vi "VSM9T_Queue_Commands.vi"(1 "VSM-9T-Control-Cluster":T1 {"Rate (T/min)" format="%6_5f"}, 3 "15T Queue":refnum<queue>) -> (0 "VSM-9T-Control-Cluster new Status":T1 {"Rate (T/min)" format="%6_5f"})   [LabVIEW 2019]
uses:
  VSM/VSM9T-Control-Cluster.ctl
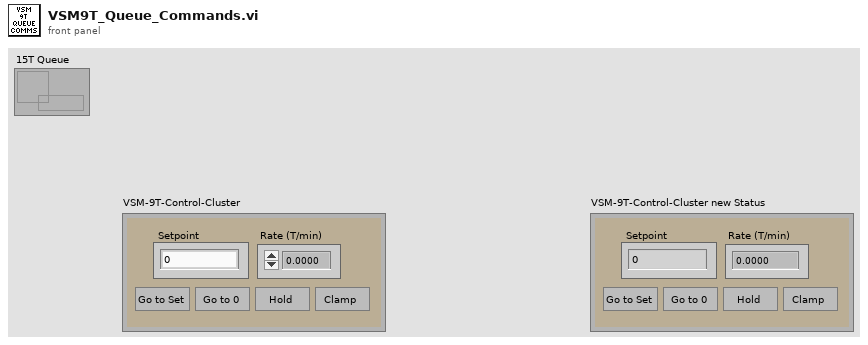
[diagram p1: front panel]
types:
  T1 = typedef "VSM9T-Control-Cluster.ctl" = cluster{"Go to set":bool, "Go to Zero":bool, "Clamp":bool, "Go to Hold":bool, "Rate (T/min)":dbl, "Setpoint":dbl}
  T2 = cluster{"Go to set":bool, "Go to Zero":bool, "Clamp":bool, "Go to Hold":bool, "Rate (T/min)":bool, "Setpoint":bool}
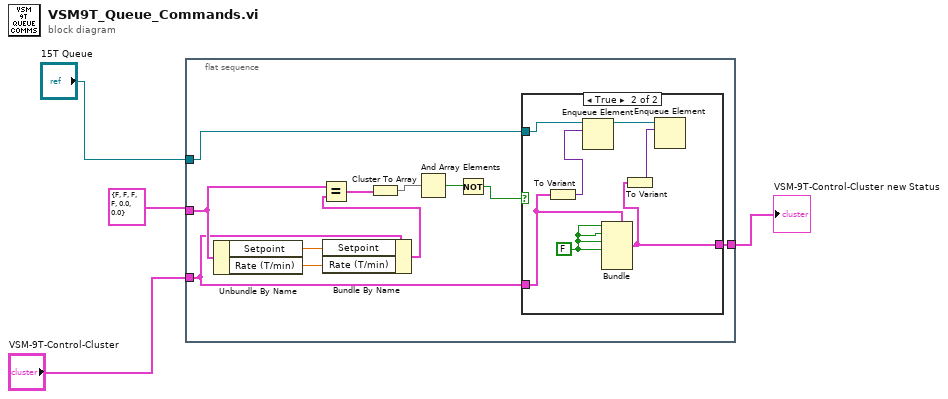
[diagram p0: block diagram]
diagram:
  n1 = flat-sequence {
    tunnel: "15T Queue" -> [w15]
    tunnel: T1 {"Go to set"=FALSE, "Go to Zero"=FALSE, "Clamp"=FALSE, "Go to Hold"=FALSE, "Rate (T/min)"=0.0, "Setpoint"=0.0} ("VSM-9T-Control-Cluster") -> [w11]
    tunnel: "VSM-9T-Control-Cluster" -> [w10]
    tunnel: [w5] -> w1
    frame #0 {
      n2 = Unbundle By Name(w11) -> ("Setpoint"=w14:dbl, "Rate (T/min)"=w13:dbl)
      n3 = Bundle By Name(cluster=w10, "Setpoint"=w14, "Rate (T/min)"=w13) -> (w12:T1)
      n4 = Equal?(x=w11, y=w12) -> (x = y?=w9:T2)
      n5 = Cluster To Array(cluster=w9) -> (array=w8:bool[])
      n6 = And Array Elements(Boolean array=w8) -> (logical AND=w7:bool)
      n7 = Not(x=w7) -> (.not. x?=w6:bool)
      n8 = case shown="True" w6 {
        tunnel: w15 -> [_ w23]
        tunnel: w10 -> [w16 w21]
        tunnel: [w16 w18] -> w5
        frame False {
        }
        frame True {
          w17 = FALSE
          n9 = To Variant(anything=w21) -> (Variant=w22:variant)
          n10 = Enqueue Element(queue=w23, element=w22) -> (queue out=w20:refnum<queue>)  [unwired: 2 in, 2 out]
          n11 = Bundle(cluster=w21, "Go to set"=w17, "Go to Zero"=w17, "Clamp"=w17, "Go to Hold"=w17) -> (w18:T1)  [unwired: 2 in]
          n12 = To Variant(anything=w18) -> (Variant=w19:variant)
          n13 = Enqueue Element(queue=w20, element=w19) -> ()  [unwired: 2 in, 3 out]
        }
      }
    }
  }
  "VSM-9T-Control-Cluster new Status" <- w1
